vi "Update_Result_Table_Value.vi"(7 "MCListbox Refnum":refnum<vi>, 8 "error in (no error)":errorcluster, 9 "AnalysisResults":variant[](array[variant]), 10 "All ROI":T1[](array[typedef]), 11 "Analysis Result":refnum<vi>) -> (0 "error out":errorcluster)   [LabVIEW 2019]
uses:
  Process/Controls/Process_Setting.ctl
  Analysis/Controls/Analysis_Setting.ctl
  Controls/Vision_DataEntry.ctl
  Analysis/Controls/V_Analysis_Type.ctl
  Ctrl/VisionProcessName.ctl
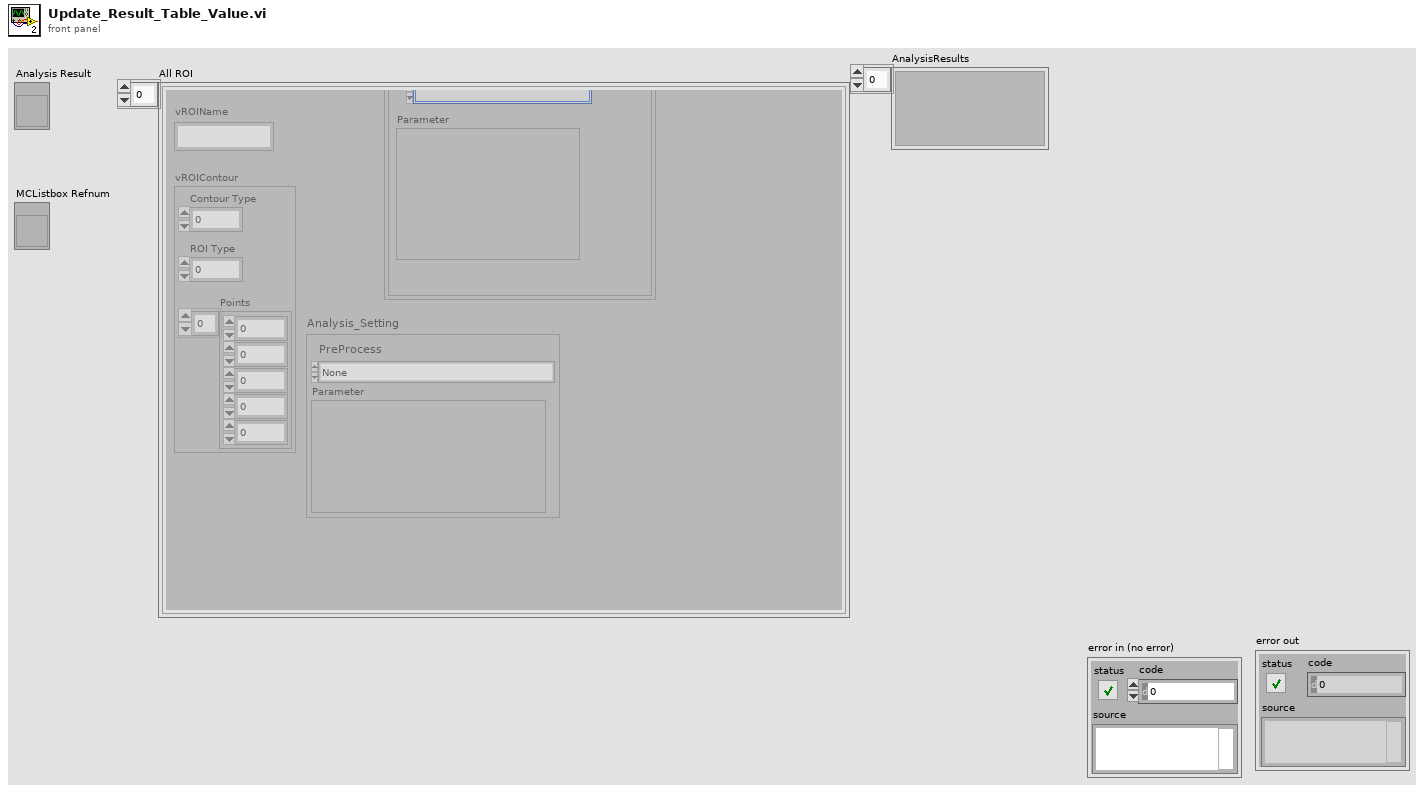
[diagram p1: front panel]
types:
  T1 = typedef "Vision_DataEntry.ctl" = cluster{"vROIName":string, "vROIContour":cluster{"Contour Type":u32, "ROI Type":u32, "Points":i32[]}, "ProcessSetting":T2[], "Analysis_Setting":T4}
  T2 = typedef "Process_Setting.ctl" = cluster{"Enum_PreProcess":T3, "Parameter":string}
  T3 = typedef "VisionProcessName.ctl" = enum16{"*CamParameter*", "CamAttributes", "*Preprocess*", "CG_Brightness", "C_Plane Extraction", "C_Threshold", "G_Lookup Table", "G_Threshold"}
  T4 = typedef "Analysis_Setting.ctl" = cluster{"PreProcess":T5, "Parameter":string}
  T5 = typedef "V_Analysis_Type.ctl" = enum16{"None", "C_Color Pattern Matching", "G_PatternMatching", "G_ShapeDectect", "G_GeometricMatch", "B_Area Check"}
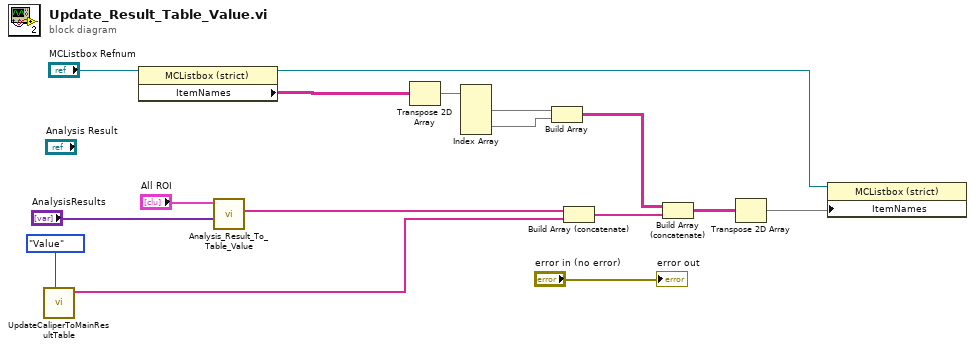
[diagram p0: block diagram]
diagram:
  n1 = call "UpdateCaliperToMainResultTable.vi"("Type"=enum16{"TagName", "Value"}."Value") -> ("CaliperResultNames"=w3:string[])  [unwired: 10 in]
  n2 = property class="MCListbox (strict)"(reference="MCListbox Refnum") -> (reference out=w11:refnum<vi>, "ItemNames"=w10:string[][])  [unwired: 1 in, 1 out]
  n3 = call "Analysis_Result_To_Table_Value.vi"("AnalysisResults"="AnalysisResults", "All ROI"="All ROI") -> ("TableValues"=w2:string[])  [unwired: 9 in]
  n4 = Transpose 2D Array(2D array=w10) -> (transposed array=w9:string[][])
  n5 = Index Array(array=w9) -> (element #1=w8:string[], element #2=w7:string[])  [unwired: 4 in]
  n6 = Build Array(w8, w7) -> (w6:string[][])
  n7 = Build Array (concatenate)(w2, w3) -> (w16:string[])
  n8 = Build Array (concatenate)(w6, w16) -> (w15:string[][])
  n9 = Transpose 2D Array(2D array=w15) -> (transposed array=w14:string[][])
  n10 = property class="MCListbox (strict)"(reference=w11, "ItemNames"=w14) -> ()  [unwired: 1 in, 2 out]
  "error out" <- "error in (no error)"
